vi "DeviceListMonitor_Main.vi"() -> ()   [LabVIEW 2020]
uses:
  Types/States.ctl
  NotifyIcon/TypeDefs/NotifyIcon Events.ctl
  NotifyIcon/TypeDefs/NotifyIcon Event Registration Actions.ctl
  <vilib>/nisyscfg/Close (System).vi
  <vilib>/addons/database/Connection.llb/DB Tools Open Connec (Path).vi
  <vilib>/regexp/Match Regular Expression.xnode
  <vilib>/nisyscfg/nisyscfg.lvlib
  <resource>/objmgr/nisysapi.rc
  <resource>/objmgr/nicontrollersysapi.rc
  <vilib>/addons/database/NI_Database_API.lvlib
panel:
  out "Time":string
  out "Current State":T1=enum."Wait"
  out "Icon Path":path
  in  "stop":bool
  out "Last error":errorcluster
  out "IP Address":string
  out "HostName":string
  out "Local Device List":string[][](table)
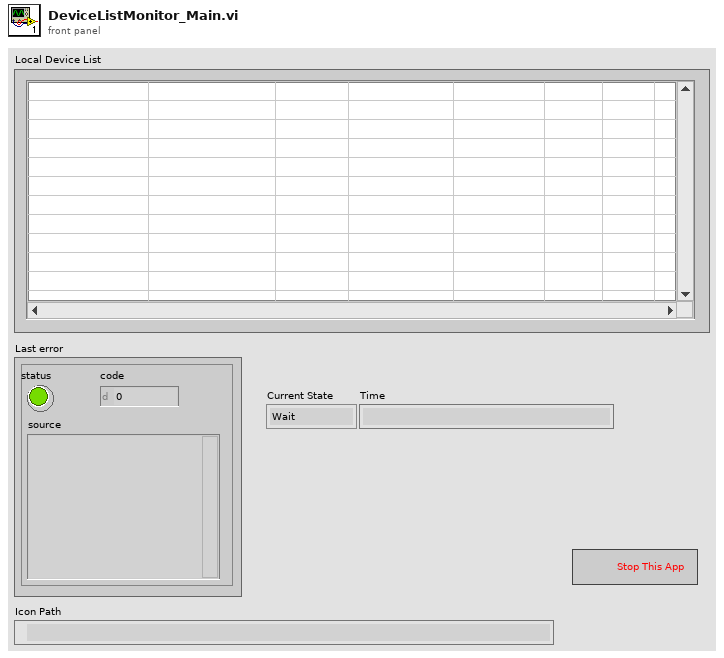
[diagram p1: front panel]
types:
  T1 = typedef "States.ctl" = enum16{"List Devices", "Log DB", "Wait"}
  T2 = enum32{"Invalid", "Standard", "Closed", "Hidden", "Minimized", "Maximized"}
  T3 = typedef "NotifyIcon Event Registration Actions.ctl" = enum16{"Initial Event Registration", "Add to Event Registration", "Destroy Events and Re-register"}
  T4 = typedef "NotifyIcon Events.ctl" = enum16{"BalloonTipClicked", "BalloonTipClosed", "BalloonTipShown", "Click", "Disposed", "DoubleClick", "MouseClick", "MouseDoubleClick", "MouseDown", "MouseMove", "MouseUp", "MenuItemClick", "MenuItemSelect"}
  T5 = typedef "NI_Database_API.lvlib/Conn ObjectReference.ctl" = refnum<k1>
  T6 = typedef "NotifyIcon Event Data.ctl" = cluster{"NotifyIcon Event":T4, "Data String":string}
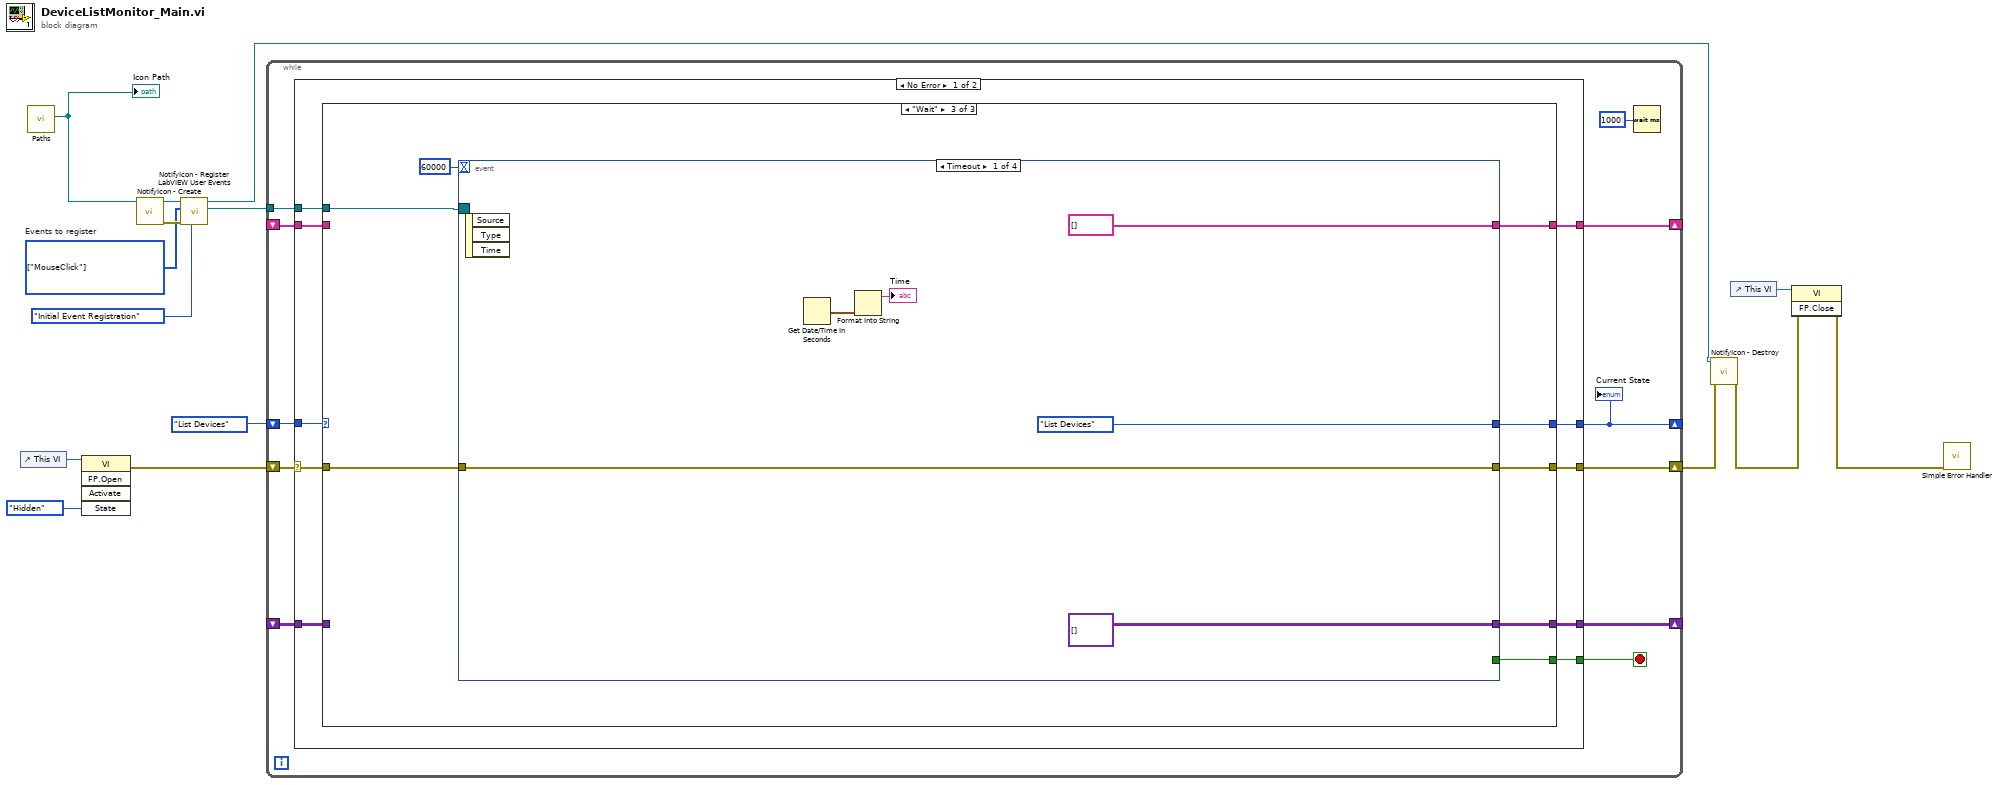
[diagram p0: block diagram]
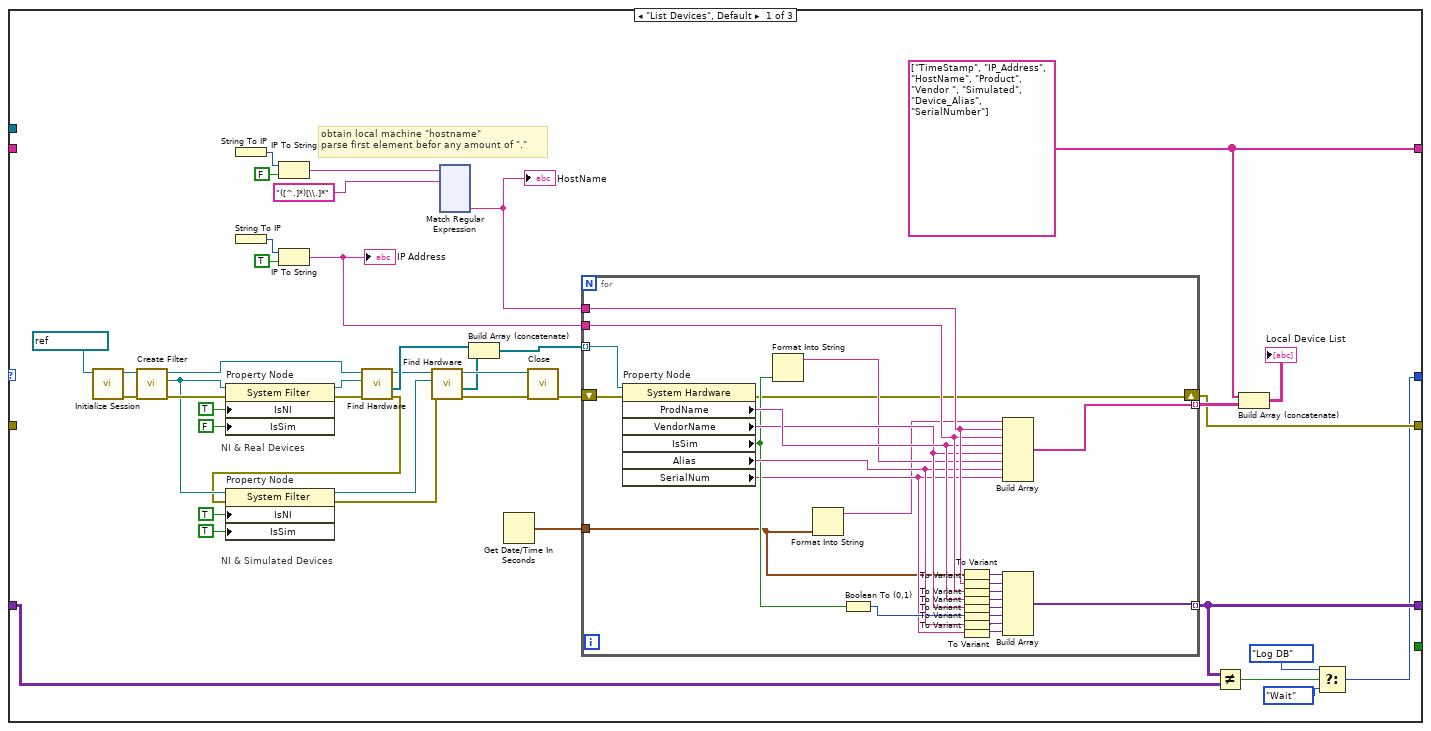
[diagram p2: hidden frame]
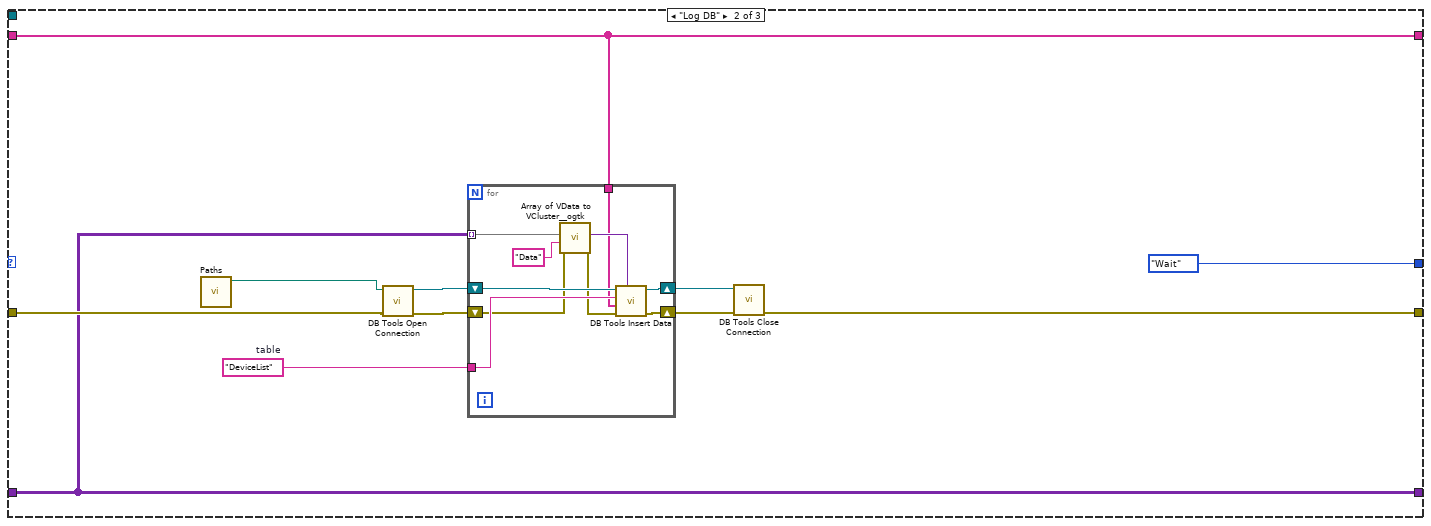
[diagram p3: hidden frame]
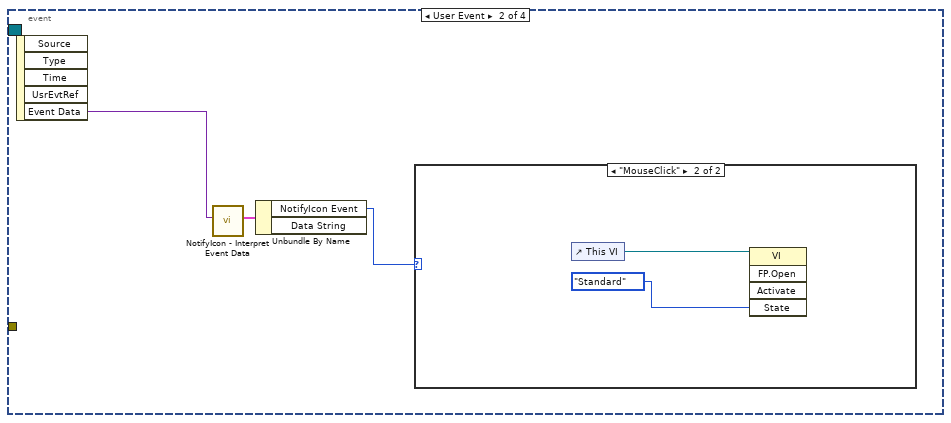
[diagram p4: hidden frame]
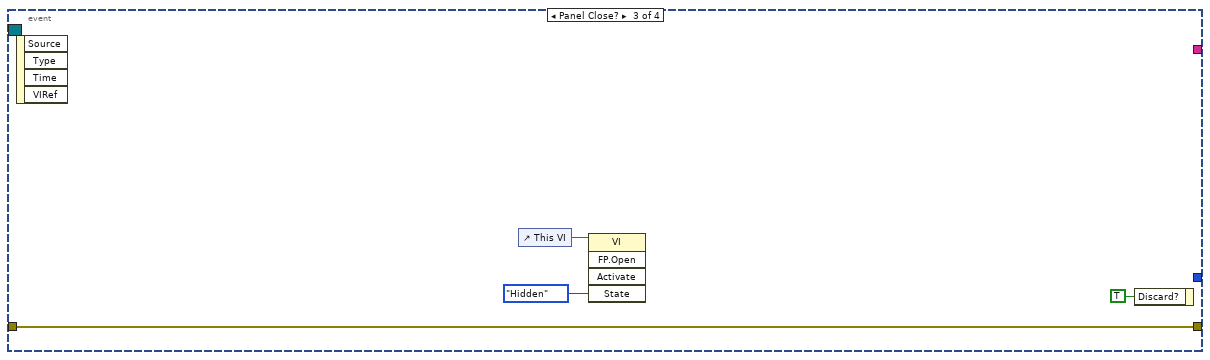
[diagram p6: hidden frame]
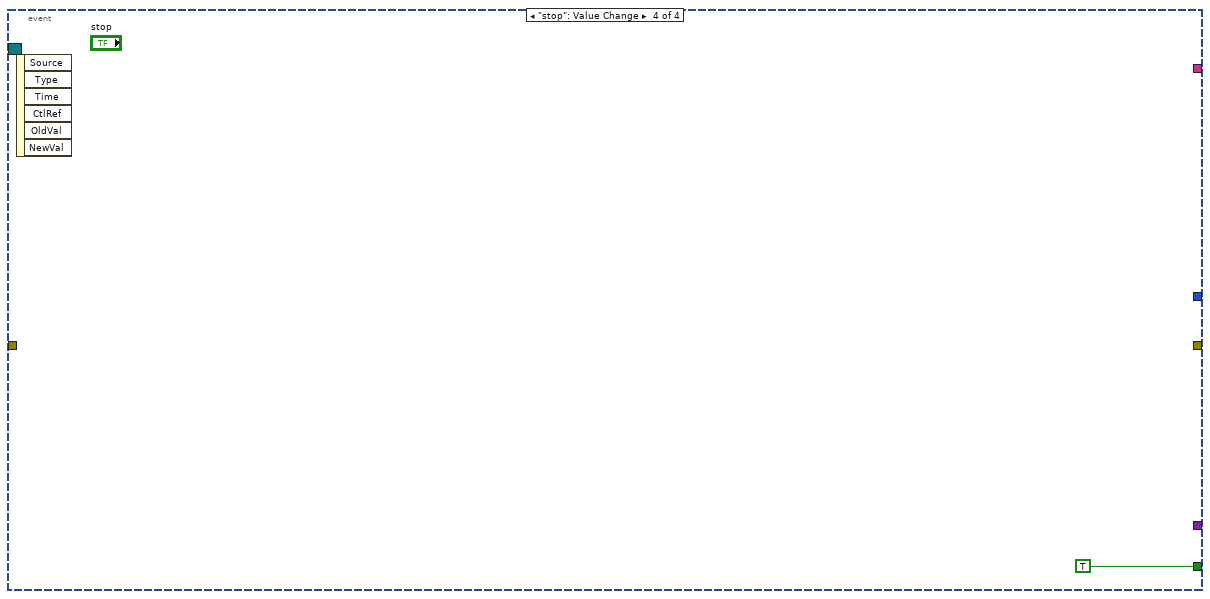
[diagram p7: hidden frame]
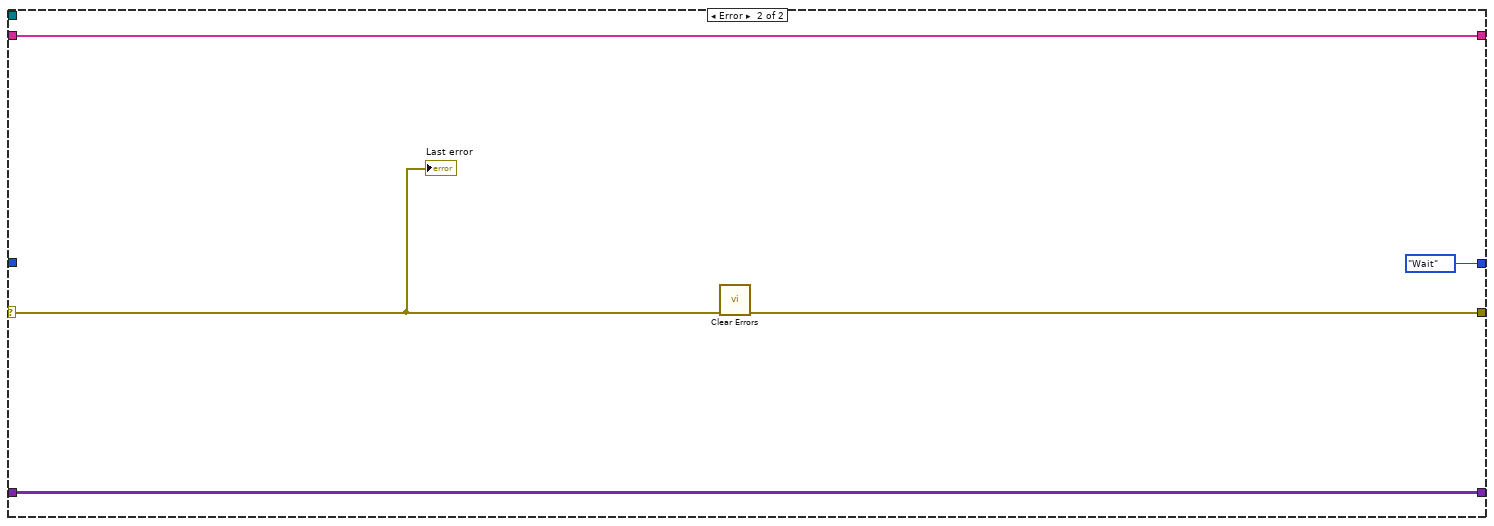
[diagram p8: hidden frame]
diagram:
  w10 = T4[] [enum."MouseClick"] items=["BalloonTipClicked", "BalloonTipClosed", "BalloonTipShown", "Click", "Disposed", "DoubleClick", "MouseClick", "MouseDoubleClick", "MouseDown", "MouseMove", "MouseUp", "MenuItemClick", "MenuItemSelect"]  # Events to register
  n1 = control-ref of="This VI"() -> (w5:refnum<vi>)
  n2 = call "Paths.vi"() -> ("Icon Path"=w9:path)  [unwired: 10 in, 1 out]
  "Icon Path" <- w9
  n3 = invoke class="VI" method="FP.Open"(reference=w5, "State"=T2."Hidden") -> (error out=w4:errorcluster)  [unwired: 3 in, 4 out]
  n4 = call "NotifyIcon - Create.vi"("Icon File Path"=w9) -> ("error out"=w14:errorcluster, "NotifyIcon reference"=w13:refnum<k24>)  [unwired: 9 in]
  n5 = call "NotifyIcon - Register LabVIEW User Events.vi"("Action"=NotifyIcon_Event_Registration_Actions."Initial Event Registration", "error in"=w14, "Events to register"=w10, "NotifyIcon reference in"=w13) -> ("Event Registration Refnum"=w11:refnum<event-registration>, "NotifyIcon reference out"=w7:refnum<k24>)  [unwired: 5 in, 1 out]
  n6 = while {
    shift-right: [w25] -> _
    shift-left: _ -> [w24]
    shift-right: [w19] -> w8
    shift-left: w4 -> [w23]
    shift-right: [w22] -> _
    shift-left: _ -> [w21]
    shift-right: [w20] -> _
    shift-left: States."List Devices" -> [w26]
    tunnel: w11 -> [w17]
    stop <- w16 stop-if-true
    n7 = case shown="No Error" w23 {
      selector: w23 -> [w33 w265]
      tunnel: w26 -> [w36 _]
      tunnel: [w35 w264] -> w25
      tunnel: w24 -> [w34 w264]
      tunnel: [w32 w263] -> w22
      tunnel: w21 -> [w31 w263]
      tunnel: [w30 States."Wait"] -> w20
      tunnel: [w29 w267] -> w19
      tunnel: w17 -> [w28 _]
      tunnel: [w27 _] -> w16
      frame No Error {
        n8 = case shown="\"Wait\"" w36 {
          tunnel: [w52 w218 w245] -> w35
          tunnel: [w56 w223 w242] -> w29
          tunnel: w34 -> [w53 w218 _]
          tunnel: w33 -> [_ w221 w243]
          tunnel: [w54 w220 w244] -> w32
          tunnel: w31 -> [_ w220 _]
          tunnel: [w48 States."Wait" w246] -> w30
          tunnel: w28 -> [_ _ w240]
          tunnel: [_ _ w239] -> w27
          frame "List Devices", Default {
            w54 = string[] ["TimeStamp", "IP_Address", "HostName", "Product", "Vendor ", "Simulated", "Device_Alias", "SerialNumber"] ("array")
            # "NI & Real Devices"
            # "NI & Simulated Devices"
            # "obtain local machine \"hostname\" \nparse first element befor any amount of \".\""
            n9 = call <vilib>:"Initialize Session.vi"("Target (localhost)"=refnum<k21> "localhost") -> ("error out"=w75:errorcluster, "Session out"=w76:refnum<k21>)  [unwired: 9 in]
            n10 = call <vilib>:"Create Filter.vi"("error in (no error)"=w75, "Session in"=w76) -> ("error out"=w77:errorcluster, "Filter out"=w40:refnum<k20>, "Session out"=w72:refnum<k21>)  [unwired: 7 in]
            n11 = property on="Property Node" class="System Filter"(reference=w40, error in=w77, "IsNI"=TRUE ("Devices & Chassis:Is NI Product"), "IsSim"=FALSE ("Devices & Chassis:Is Simulated")) -> (reference out=w73:refnum<k20>, error out=w74:errorcluster)
            n12 = String To IP() -> (0:w64:u32)  [unwired: 1 in]
            n13 = String To IP() -> (0:w60:u32)  [unwired: 1 in]
            n14 = IP To String(1:FALSE ("dot notation? (F)"), 2:w64) -> (0:w65:string)
            n15 = IP To String(1:TRUE ("dot notation? (F)"), 2:w60) -> (0:w59:string)
            "IP Address" <- w59
            n16 = call <vilib>:"Find Hardware.vi"("error in (no error)"=w74, "Filter in"=w73, "Session in"=w72) -> ("error out"=w38:errorcluster, "Resources out"=w70:refnum<k20>[], "Session out"=w47:refnum<k21>)  [unwired: 5 in, 1 out]
            n17 = property on="Property Node" class="System Filter"(reference=w40, error in=w38, "IsNI"=TRUE ("Devices & Chassis:Is NI Product"), "IsSim"=TRUE ("Devices & Chassis:Is Simulated")) -> (reference out=w39:refnum<k20>, error out=w37:errorcluster)
            n18 = call <vilib>:"Find Hardware.vi"("error in (no error)"=w37, "Filter in"=w39, "Session in"=w47) -> ("error out"=w46:errorcluster, "Resources out"=w43:refnum<k20>[], "Session out"=w45:refnum<k21>)  [unwired: 5 in, 1 out]
            n19 = xnode "Match Regular Expression"("input string"=w65, "regular expression"="([^.]*)[\\.]*") -> ("submatch 1"=w58:string)  [unwired: 4 in, 5 out]
            "HostName" <- w58
            n20 = Build Array (concatenate)(w70, w43) -> (w44:refnum<k20>[])
            n21 = Get Date/Time In Seconds() -> (seconds since 1Jan1904=w57:timestamp)
            n22 = call-poly <vilib>:"Close.vi"("error in (no error)"=w46, "Session in"=w45) -> ("error out"=w69:errorcluster)  [unwired: 9 in]
            n23 = for {
              tunnel: w44 -> [w216] mode=indexing
              tunnel: [w215] -> w68 mode=indexing
              tunnel: w59 -> [w206]
              tunnel: w58 -> [w207]
              tunnel: w57 -> [w196]
              tunnel: [w195] -> w52 mode=indexing
              shift-right: [w194] -> w56
              shift-left: w69 -> [w217]
              n24 = property on="Property Node" class="System Hardware"(reference=w216, error in=w217) -> (error out=w194:errorcluster, "ProdName"=w205:string, "VendorName"=w204:string, "IsSim"=w201:bool, "Alias"=w202:string, "SerialNum"=w198:string)  [unwired: 1 out]
              n25 = Format Into String "Format Into String"(w201) -> (resulting string=w203:string)  [unwired: 3 in, 1 out]
              n26 = Format Into String "Format Into String"(w196) -> (resulting string=w197:string)  [unwired: 3 in, 1 out]
              n27 = Boolean To (0,1)(Boolean=w201) -> (0, 1=w200:i16)
              n28 = To Variant(anything=w196) -> (Variant=w214:variant)
              n29 = To Variant(anything=w207) -> (Variant=w213:variant)
              n30 = To Variant(anything=w206) -> (Variant=w212:variant)
              n31 = To Variant(anything=w205) -> (Variant=w211:variant)
              n32 = To Variant(anything=w204) -> (Variant=w210:variant)
              n33 = To Variant(anything=w200) -> (Variant=w209:variant)
              n34 = To Variant(anything=w202) -> (Variant=w208:variant)
              n35 = To Variant(anything=w198) -> (Variant=w199:variant)
              n36 = Build Array "Build Array"(w197, w207, w206, w205, w204, w203, w202, w198) -> (w215:string[])
              n37 = Build Array "Build Array"(w214, w213, w212, w211, w210, w209, w208, w199) -> (w195:variant[])
            }
            n38 = Not Equal?(x=w52, y=w53) -> (x != y?=w51:bool)
            n39 = Build Array (concatenate)(w54, w68) -> (→"Local Device List":string[][])
            n40 = Select(t=States."Log DB", s=w51, f=States."Wait") -> (s? t:f=w48:T1)
          }
          frame "Log DB" {
            w224 = "DeviceList"  # table
            n41 = call "Paths.vi"() -> ("UDL Path"=w225:path)  [unwired: 10 in, 1 out]
            n42 = call-poly <vilib>:"DB Tools Open Connection.vi"("error in (no error)"=w221, "connection information"=w225) -> ("error out"=w222:errorcluster, "connection reference"=w226:T5)  [unwired: 6 in]
            n43 = for {
              tunnel: w224 -> [w234]
              tunnel: w218 -> [w233] mode=indexing
              shift-right: [w238] -> w228
              shift-left: w226 -> [w236]
              shift-right: [w237] -> w227
              shift-left: w222 -> [w231]
              tunnel: w220 -> [w229]
              n44 = call <userlib>:"Array of VData to VCluster__ogtk.vi"("error in (no error)"=w231, "Cluster Name"="Data", "Array"=w233) -> ("error out"=w230:errorcluster, "VCluster"=w232:variant)  [unwired: 7 in]
              n45 = call <vilib>:"DB Tools Insert Data.vi"("data"=w232, "error in (no error)"=w230, "columns"=w229, "table"=w234, "connection reference"=w236) -> ("error out"=w237:errorcluster, "connection reference out"=w238:T5)  [unwired: 5 in]
            }
            n46 = call <vilib>:"DB Tools Close Connection.vi"("error in (no error)"=w227, "connection reference"=w228) -> ("error out"=w223:errorcluster)  [unwired: 5 in]
          }
          frame "Wait" {
            n47 = event shown="[0] Timeout" {
              selector: w240 -> [_ _ _ _]
              dyn-events: _ -> [_ _ _ _]
              timeout: 60000 -> [_ _ _ _]
              tunnel: [States."List Devices" _ _ _] -> w246
              tunnel: [variant[][] [] _ _ _] -> w245
              tunnel: [string[] [] ("array") _ _ _] -> w244
              tunnel: w243 -> [w249 _ w260 _]
              tunnel: [w249 _ w260 _] -> w242
              tunnel: [_ _ _ TRUE] -> w239
              event Timeout {
                n48 = event-data() -> ()  [unwired: 1 in, 3 out]
                n49 = Get Date/Time In Seconds() -> (seconds since 1Jan1904=w248:timestamp)
                n50 = Format Into String(w248) -> (resulting string=→"Time":string)  [unwired: 3 in, 1 out]
              }
              event User Event {
                n51 = event-data() -> ("Event Data"=w254:variant)  [unwired: 1 in, 4 out]
                n52 = call "NotifyIcon - Interpret Event Data.vi"("NotifyIcon Event Data"=w254) -> ("NotifyIcon Event Data"=w255:T6)  [unwired: 9 in, 1 out]
                n53 = Unbundle By Name(w255) -> ("NotifyIcon Event"=w253:T4)  [unwired: 1 out]
                n54 = case shown="\"MouseClick\"" w253 {
                  frame "BalloonTipClicked", Default {
                  }
                  frame "MouseClick" {
                    n55 = control-ref of="This VI"() -> (w257:refnum<vi>)
                    n56 = invoke class="VI" method="FP.Open"(reference=w257, "State"=T2."Standard" ("Front Panel Window:State")) -> ()  [unwired: 3 in, 5 out]
                  }
                }
              }
              event Panel Close? {
                n57 = event-data() -> ()  [unwired: 1 in, 4 out]
                n58 = control-ref of="This VI"() -> (w259:refnum<vi>)
                n59 = invoke class="VI" method="FP.Open"(reference=w259, "State"=T2."Hidden") -> ()  [unwired: 3 in, 5 out]
                n60 = event-data("Discard?"=TRUE) -> ()  [unwired: 1 in, 1 out]
              }
              event "stop": Value Change {
                n61 = event-data() -> ()  [unwired: 1 in, 6 out]
              }
            }
          }
        }
      }
      frame Error {
        n62 = call <vilib>:"Clear Errors.vi"("error in (no error)"=w265) -> ("error out"=w267:errorcluster)  [unwired: 5 in, 1 out]
        "Last error" <- w265
      }
    }
    "Current State" <- w20
    n63 = Wait (ms)(milliseconds to wait=u32 1000) -> ()  [unwired: 1 out]
  }
  n64 = call "NotifyIcon - Destroy.vi"("error in"=w8, "NotifyIcon reference"=w7) -> ("error out"=w2:errorcluster)  [unwired: 9 in]
  n65 = control-ref of="This VI"() -> (w3:refnum<vi>)
  n66 = invoke class="VI" method="FP.Close"(reference=w3, error in=w2) -> (error out=w1:errorcluster)  [unwired: 1 in, 2 out]
  n67 = call <vilib>:"Simple Error Handler.vi"("error in (no error)"=w1) -> ()  [unwired: 4 in, 5 out]
